vi "updateConfiguration.vi"(8 "error in (no error)":errorcluster, 9 "data":string, 10 "dataName":string, 11 "ConfigurationFileReader in":refnum<class "ConfigurationFileReader.lvclass">) -> (0 "error out":errorcluster, 3 "ConfigurationFileReader out":refnum<class "ConfigurationFileReader.lvclass">)   [LabVIEW 2016, in "Settings.lvlib" / "ConfigurationFileReader.lvclass"]
doc: "Writes data to a configuration file."
uses:
  ConfigurationFileReader.lvclass
  <vilib>/Utility/xml.llb/Write to XML File(string).vi
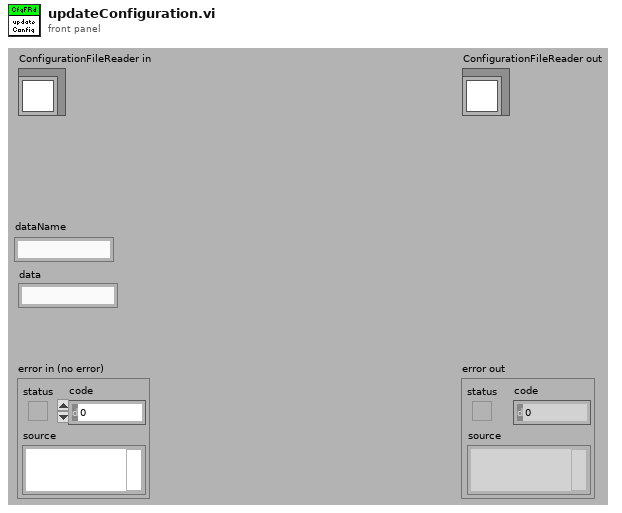
[diagram p1: front panel]
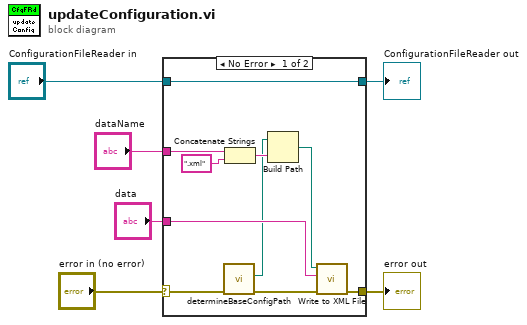
[diagram p0: block diagram]
diagram:
  n1 = case shown="No Error" "error in (no error)" {
    selector: "error in (no error)" -> [w9 w18]
    tunnel: [w14 w18] -> w5
    tunnel: [w16 w17] -> w3
    tunnel: "ConfigurationFileReader in" -> [w16 w17]
    tunnel: "dataName" -> [w15 _]
    tunnel: "data" -> [w12 _]
    frame No Error {
      n2 = call "determineBaseConfigPath.vi"("error in (no error)"=w9) -> ("error out"=w8:errorcluster, "baseConfigPath"=w7:path)  [unwired: 8 in, 1 out]
      n3 = Concatenate Strings(w15, ".xml" ("string")) -> (w11:string)
      n4 = Build Path(base path=w7, name or relative path=w11) -> (appended path=w10:path)
      n5 = call-poly <vilib>:"Write to XML File.vi"("error in (no error)"=w8, "XML Input"=w12, "XML File Path"=w10) -> ("error out"=w14:errorcluster)  [unwired: 6 in, 2 out]
    }
    frame Error {
    }
  }
  "error out" <- w5
  "ConfigurationFileReader out" <- w3
